vi "capex digital ttl.vi"() -> ()   [LabVIEW 2013]
uses:
  <vilib>/Waveform/DWDTOps.llb/DWDT Boolean Array to Digital.vi
  <vilib>/Waveform/DTblOps.llb/DTbl Digital to Boolean Array.vi
panel:
  in  "stop":bool
  in  "GPIO registers set":digitaldata={"transitions"=[], "data"=[[0, 0, 0, 0, 0, 0, 0, 0, 0, 0, 0, 0, 0, 0, 0, 0, 0, 0, 0, 0, 0, 0, 0, 0, 0, 0, 0, 0, 0, 0, 0, 0]]}
  in  "Execute update":bool
  out "GPIO registers read":digitaldata
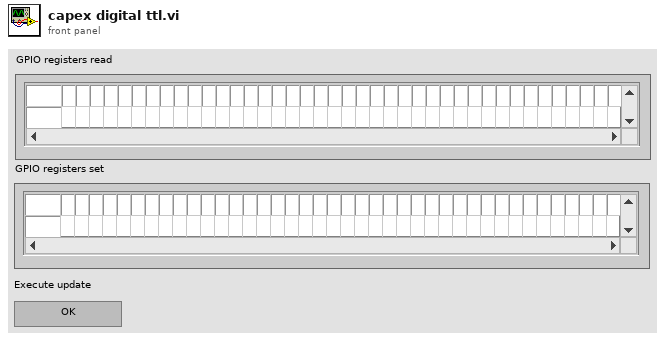
[diagram p1: front panel]
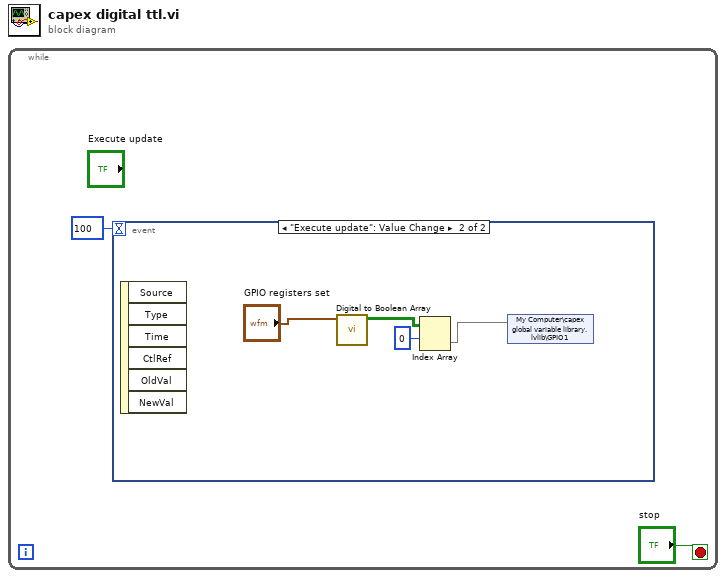
[diagram p0: block diagram]
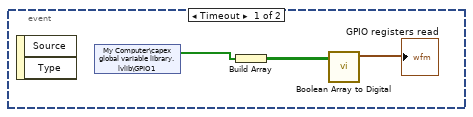
[diagram p2: hidden frame]
diagram:
  n1 = while {
    stop <- "stop" stop-if-true
    n2 = event shown="[1] \"Execute update\": Value Change" {
      selector: _ -> [_ _]
      dyn-events: _ -> [_ _]
      timeout: 100 -> [_ _]
      event Timeout {
        n3 = event-data() -> ()  [unwired: 1 in, 2 out]
        n4 = shared-variable "My Computer\\capex global variable library.lvlib\\GPIO1"() -> (w4:bool[])  [unwired: 1 in, 1 out]
        n5 = Build Array(w4) -> (w3:bool[][])
        n6 = call-poly <vilib>:"Boolean Array to Digital.vi"("boolean array"=w3) -> ("digital waveform"=→"GPIO registers read":digitalwaveform)  [unwired: 9 in, 1 out]
      }
      event "Execute update": Value Change {
        n7 = event-data() -> ()  [unwired: 1 in, 6 out]
        n8 = call-poly <vilib>:"Digital to Boolean Array.vi"("digital data"="GPIO registers set") -> ("boolean array"=w8:bool[][])  [unwired: 9 in, 1 out]
        n9 = Index Array(array=w8, index (row)=0) -> (element=w7:bool[])  [unwired: 1 in]
        n10 = shared-variable "My Computer\\capex global variable library.lvlib\\GPIO1"(w7) -> ()  [unwired: 1 in, 1 out]
      }
    }
  }
